vi "Set Tickbox Caption.vi"(8 "Error In":errorcluster, 10 "Caption":string, 11 "Tickbox Ref":refnum<vi>) -> (0 "Error Out":errorcluster)   [LabVIEW 2022 SP3]
doc: "<add documentation here>"
panel:
  # "Development\nControls or indicators that are useful for development or testing, but which are not outputs of the VI."
  # "Input\nInputs to the VI"
  # "Output\nOutputs of the VI"
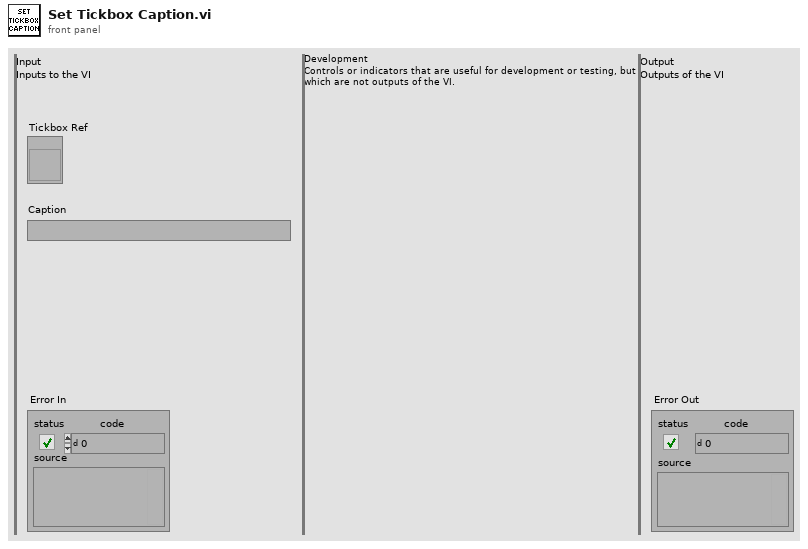
[diagram p1: front panel]
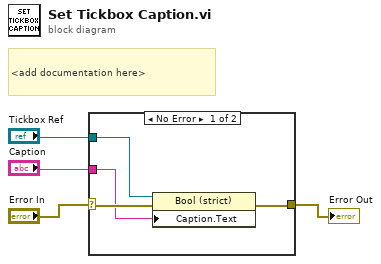
[diagram p0: block diagram]
diagram:
  # "<add documentation here>"
  n1 = case shown="No Error" "Error In" {
    selector: "Error In" -> [w8 w9]
    tunnel: [w7 w9] -> w3
    tunnel: "Tickbox Ref" -> [w6 _]
    tunnel: "Caption" -> [w5 _]
    frame No Error {
      n2 = property class="Bool (strict)"(reference=w6, error in=w8, "Caption.Text"=w5) -> (error out=w7:errorcluster)  [unwired: 1 out]
    }
    frame Error {
    }
  }
  "Error Out" <- w3
